vi "Get Data.vi"(8 "error in":errorcluster, 11 "AlicatMData in":refnum<class "AlicatMCData.lvclass">) -> (0 "error out":errorcluster, 2 "SystemData":T1, 3 "AlicatMData out":refnum<class "AlicatMCData.lvclass">)   [LabVIEW 2015, in "Alicat.lvlib" / "AlicatMCData.lvclass"]
doc: "Convert the data from a generic data object to something meaningful for an M/MC series Alicat device."
uses:
  AlicatMCData.lvclass
  AlicatMCData.lvclass/AlicatMCData.ctl
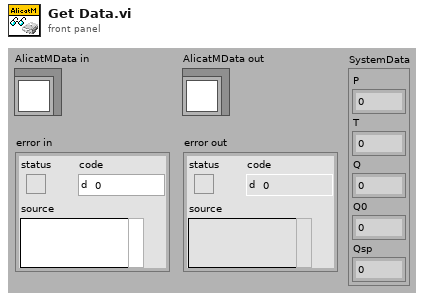
[diagram p1: front panel]
types:
  T1 = cluster{"P":sgl, "T":sgl, "Q":sgl, "Q0":sgl, "Qsp":sgl}
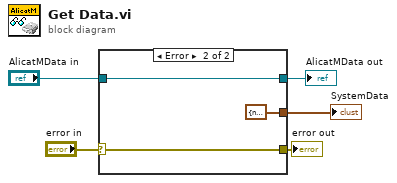
[diagram p0: block diagram]
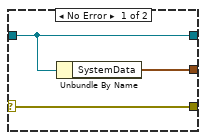
[diagram p2: hidden frame]
diagram:
  n1 = case shown="Error" "error in" {
    selector: "error in" -> [w8 w11]
    tunnel: [w8 w11] -> w4
    tunnel: [w7 w10] -> w2
    tunnel: "AlicatMData in" -> [w7 w10]
    tunnel: [w6 T1 {"P"=nan, "T"=nan, "Q"=nan, "Q0"=nan, "Qsp"=nan} ("SystemData")] -> w1
    frame No Error {
      n2 = Unbundle By Name(w7) -> ("SystemData"=w6:T1)
    }
    frame Error {
    }
  }
  "error out" <- w4
  "AlicatMData out" <- w2
  "SystemData" <- w1
